vi "init_Network Stream.vi"(8 "error in":errorcluster, 11 "MyRIO IP Address":string="172.22.11.2") -> (0 "error out":errorcluster, 3 "reader":refnum<k21>)   [LabVIEW 2019]
doc: "This VI initialize the network stream part."
uses:
  ROVdataOut.ctl
panel:
  # "This VI initialize the network stream part."
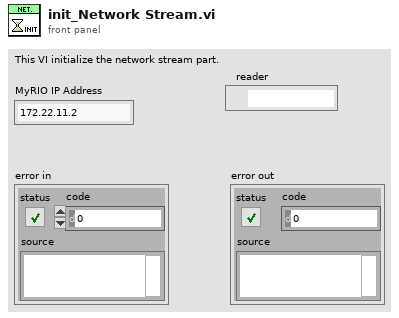
[diagram p1: front panel]
types:
  T1 = typedef "ROVdataOut.ctl" = cluster{"Rotation Angle":dbl, "Rotation Vector":cluster{"x":dbl, "y":dbl, "z":dbl}, "PING A distance":dbl, "Ping B distance":dbl, "angles":cluster{"roll":dbl, "pitch":dbl, "yaw":dbl}}
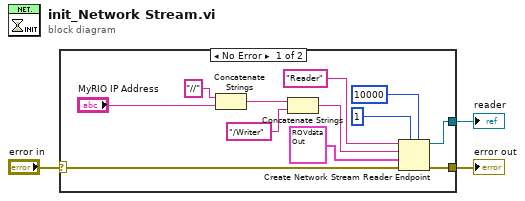
[diagram p0: block diagram]
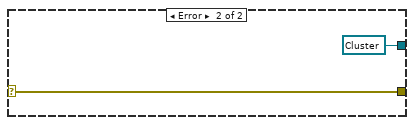
[diagram p2: hidden frame]
diagram:
  n1 = case shown="No Error" "error in" {
    selector: "error in" -> [w8 w17]
    tunnel: [w7 refnum<k21> refnum ("reader endpoint")] -> w1
    tunnel: [w6 w17] -> w2
    frame No Error {
      n2 = Concatenate Strings("//" ("reader url"), "MyRIO IP Address") -> (w12:string)
      n3 = Concatenate Strings(w12, "/Writer" ("reader url")) -> (w13:string)
      n4 = Create Network Stream Reader Endpoint(5:10000 ("timeout in ms (-1)"), 7:1 ("reader buffer size"), 8:w8, 9:T1 {"Rotation Angle"=0.0, "Rotation Vector"={"x"=0.0, "y"=0.0, "z"=0.0}, "PING A distance"=0.0, "Ping B distance"=0.0, "angles"={"roll"=0.0, "pitch"=0.0, "yaw"=0.0}} ("Cluster"), 10:w13, 11:"Reader" ("writer name")) -> (0:w6:errorcluster, 3:w7:refnum<k21>)  [unwired: 1 in]
    }
    frame Error {
    }
  }
  "error out" <- w2
  "reader" <- w1
